vi "InitSingleDevice.vi"(4 "error in (no error)":errorcluster, 6 "msecDelayForDiscovery":i32, 7 "logging":bool) -> (0 "error out":errorcluster, 2 "DeviceKey Out":string, 3 "CmdLib Out":refnum<k24>)   [LabVIEW 2009]
uses:
  C:/Code/Apps/Utilities/Picomotor/PicomotorApp/Install/Samples/LabVIEW/Model 8743/LabVIEW 2009/CmdLib.dll
panel:
  in  "deviceKey":string
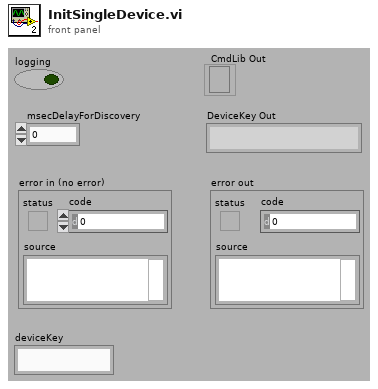
[diagram p1: front panel]
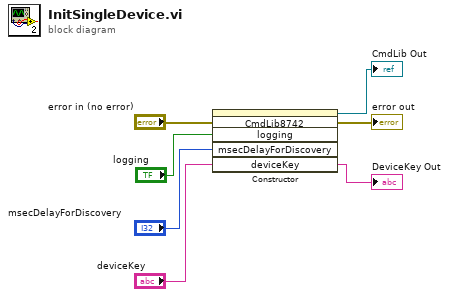
[diagram p0: block diagram]
diagram:
  n1 = constructor class="CmdLib8742"(error in="error in (no error)", "logging"="logging", "msecDelayForDiscovery"="msecDelayForDiscovery", "deviceKey"="deviceKey") -> (reference out=→"CmdLib Out":refnum<k24>, error out=→"error out":errorcluster, "deviceKey"=→"DeviceKey Out":string)  [unwired: 2 in, 3 out]
